vi "Replace DLU.vi"(8 "error in":errorcluster, 10 "Replacement VI":path, 11 "Current Bus Path":path) -> (0 "error out":errorcluster)   [LabVIEW 2014]
uses:
  <vilib>/Utility/traverseref.llb/TRef TravTarget.ctl
  <vilib>/Utility/traverseref.llb/VI Scripting - Traverse.lvlib
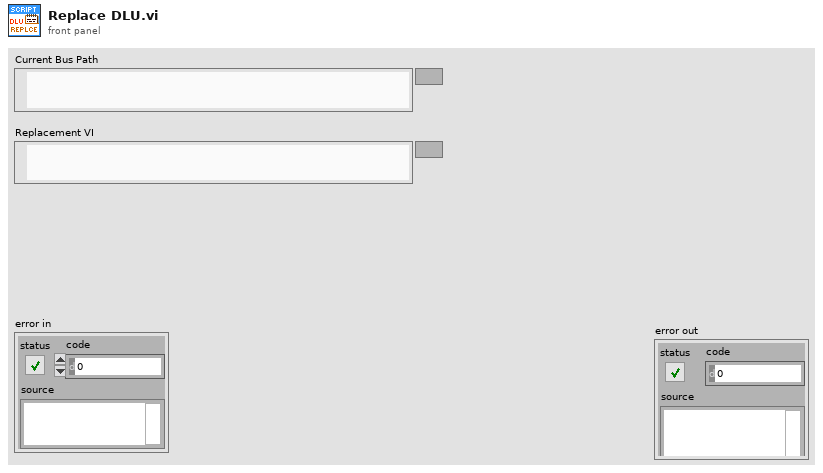
[diagram p1: front panel]
types:
  T1 = typedef "TRef TravTarget.ctl" = enum16{"FP", "BD", "Other"}
  T2 = enum32{"Invalid", "Standard", "Closed", "Hidden", "Minimized", "Maximized"}
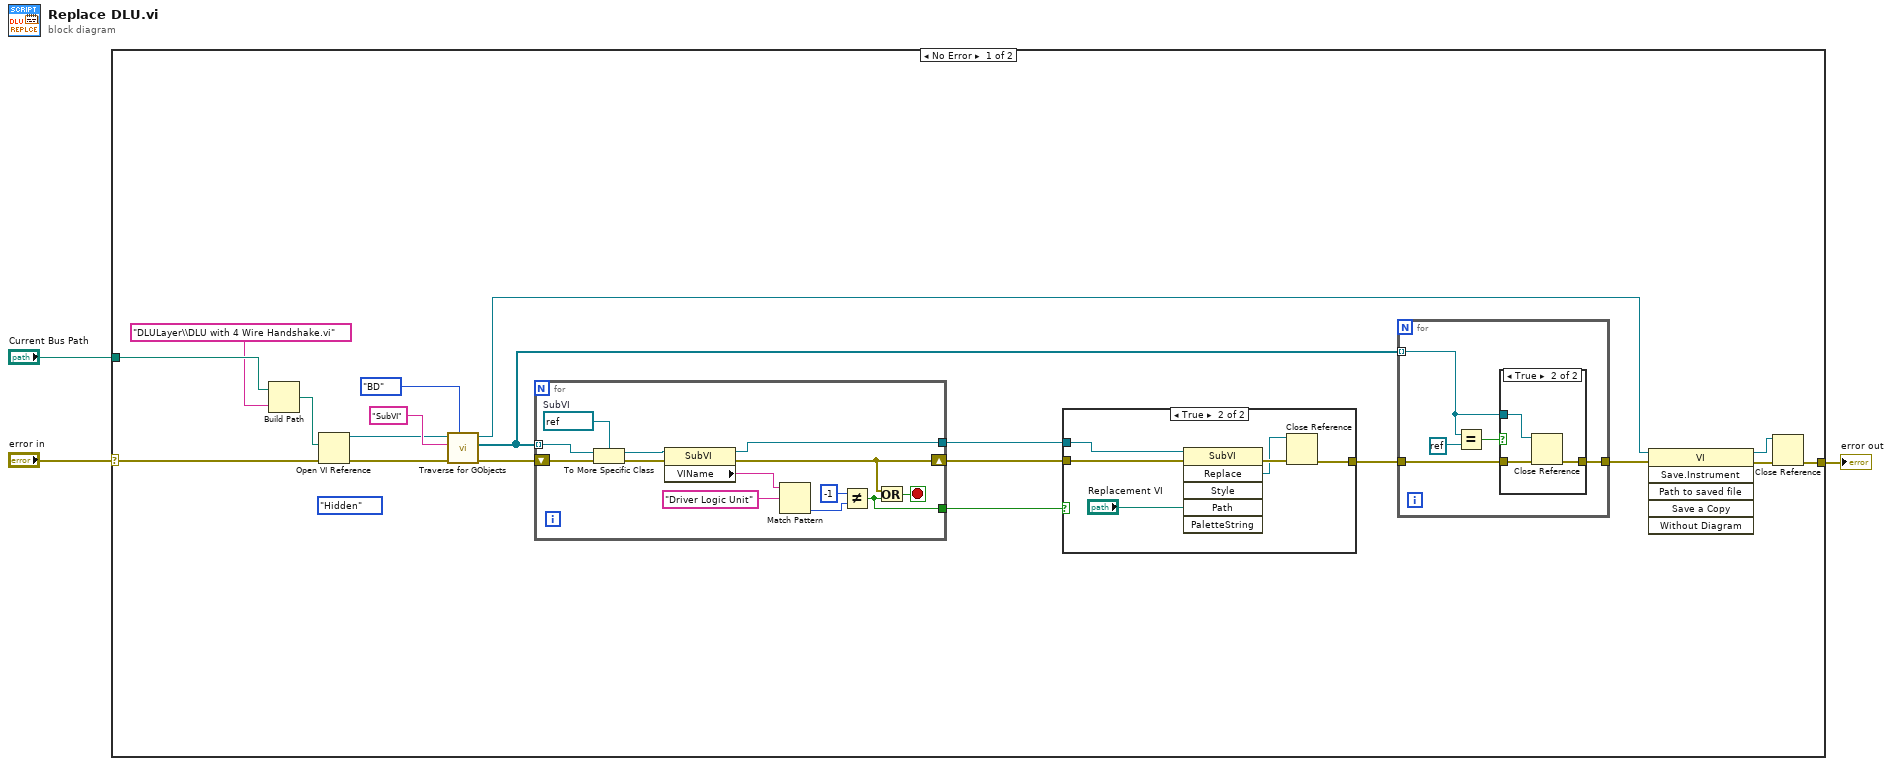
[diagram p0: block diagram]
diagram:
  n1 = case shown="No Error" "error in" {
    selector: "error in" -> [w22 w52]
    tunnel: "Current Bus Path" -> [w18 _]
    tunnel: [w6 w52] -> w1
    frame No Error {
      (unwired) T2."Hidden" ("State")
      n2 = Build Path(base path=w18, name or relative path="DLULayer\\DLU with 4 Wire Handshake.vi") -> (appended path=w21:path)
      n3 = Open VI Reference(vi path=w21, error in (no error)=w22) -> (vi reference=w9:refnum<vi>, error out=w10:errorcluster)  [unwired: 4 in]
      n4 = call <vilib>:"Traverse for GObjects.vi"("Traverse Target"=TRef_TravTarget."BD", "error in (no error)"=w10, "Class Name"="SubVI", "VI Refnum"=w9) -> ("error out"=w16:errorcluster, "References"=w11:refnum<vi>[], "dup VI Refnum"=w7:refnum<vi>)  [unwired: 4 in, 1 out]
      n5 = for {
        tunnel: w11 -> [w51] mode=indexing
        shift-right: [w45] -> w13
        shift-left: w16 -> [w49]
        tunnel: [w44] -> w15
        tunnel: [w43] -> w14
        stop <- w46 stop-if-true
        w50 = refnum<vi> refnum  # SubVI
        n6 = To More Specific Class(target class=w50, reference=w51, error in=w49) -> (specific class reference=w48:refnum<vi>, error out=w47:errorcluster)
        n7 = property class="SubVI"(reference=w48, error in=w47) -> (reference out=w43:refnum<vi>, error out=w45:errorcluster, "VIName"=w41:string)
        n8 = Match Pattern(string=w41, regular expression="Driver Logic Unit" ("y")) -> (offset past match=w40:i32)  [unwired: 1 in, 3 out]
        n9 = Not Equal?(x=-1, y=w40) -> (x != y?=w44:bool)
        n10 = Or(x=w45, y=w44) -> (x .or. y?=w46:bool)
      }
      n11 = case shown="True" w15 {
        tunnel: w14 -> [_ w38]
        tunnel: w13 -> [w32 w37]
        tunnel: [w32 w33] -> w12
        frame False {
        }
        frame True {
          n12 = invoke class="SubVI" method="Replace"(reference=w38, error in=w37, "Path"="Replacement VI") -> (error out=w35:errorcluster, "Replace"=w34:refnum<vi>)  [unwired: 3 in, 4 out]
          n13 = Close Reference(reference=w34, error in (no error)=w35) -> (error out=w33:errorcluster)
        }
      }
      n14 = for {
        tunnel: w12 -> [w27]
        tunnel: [w26] -> w8
        tunnel: w11 -> [w23] mode=indexing
        n15 = Equal?(x=w23, y=refnum<k0> refnum) -> (x = y?=w24:bool)
        n16 = case shown="True" w24 {
          tunnel: w27 -> [w28 w31]
          tunnel: [w28 w30] -> w26
          tunnel: w23 -> [_ w29]
          frame False {
          }
          frame True {
            n17 = Close Reference(reference=w29, error in (no error)=w31) -> (error out=w30:errorcluster)
          }
        }
      }
      n18 = invoke class="VI" method="Save.Instrument"(reference=w7, error in=w8) -> (reference out=w4:refnum<vi>, error out=w5:errorcluster)  [unwired: 4 in, 4 out]
      n19 = Close Reference(reference=w4, error in (no error)=w5) -> (error out=w6:errorcluster)
    }
    frame Error {
    }
  }
  "error out" <- w1
